vi "Wait.vi"(10 "Error In":errorcluster, 11 "Seconds":dbl=4.0) -> (2 "Error Out":errorcluster)   [LabVIEW 2020]
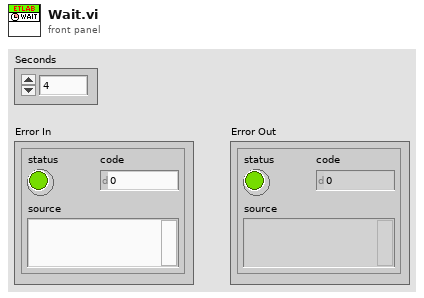
[diagram p1: front panel]
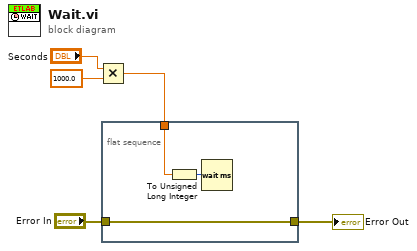
[diagram p0: block diagram]
diagram:
  n1 = Multiply(x="Seconds", y=1000.0 ("millisecond multiple")) -> (x*y=w5:dbl)
  n2 = flat-sequence {
    tunnel: w5 -> [w6]
    tunnel: "Error In" -> [w8]
    tunnel: [w8] -> w1
    frame #0 {
      n3 = To Unsigned Long Integer(number=w6) -> (unsigned 32bit integer=w7:u32)
      n4 = Wait (ms)(milliseconds to wait=w7) -> ()  [unwired: 1 out]
    }
  }
  "Error Out" <- w1
